vi "TSI Single Socket C-V Sweep SData Ver1.0.vi"(0 "Base Path":path=path "C:/Andy Tr/Wafer Level Measurement/WS102x", 1 "Package":string, 2 "Data In":string[][](array[string]), 3 "TP":string, 4 "Cyc":string, 5 "Cell":string, 7 "VDD To PGR OTP":string, 9 "Lot":string="Test", 10 "Index":i32, 11 "error in (no error)":errorcluster, 12 "Wafer":string="T8", 13 "X":string, 14 "Y":string) -> (15 "error out":errorcluster)   [LabVIEW 2017]
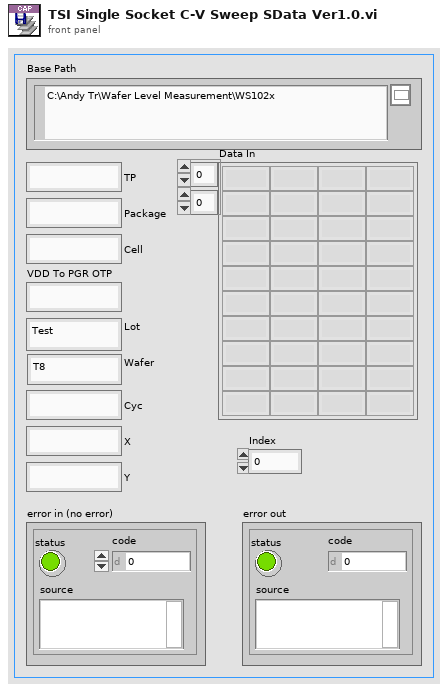
[diagram p1: front panel]
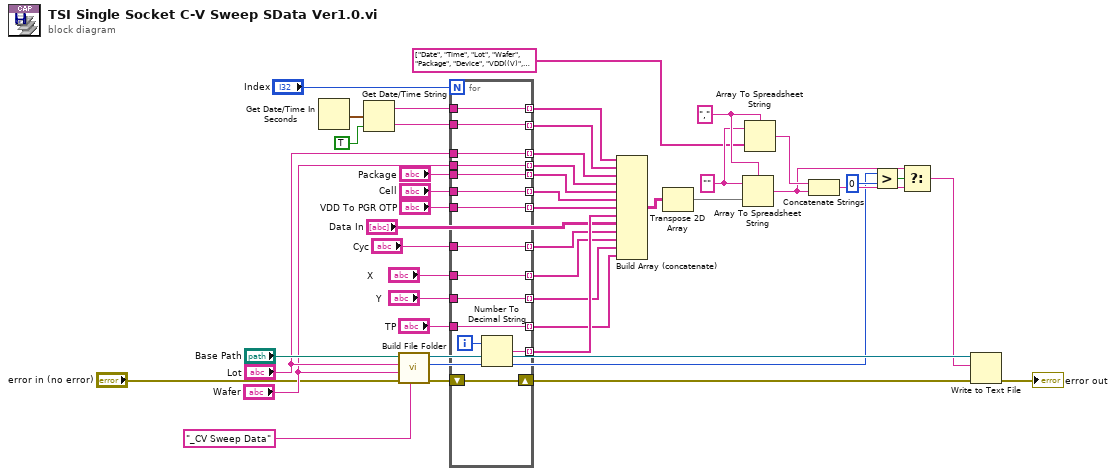
[diagram p0: block diagram]
diagram:
  w29 = "," ("delimiter (Tab)")
  w28 = "" ("format string")
  n1 = Get Date/Time In Seconds() -> (seconds since 1Jan1904=w41:timestamp)
  n2 = Get Date/Time String(seconds (now)=w41, want seconds? (F)=TRUE) -> (date string=w40:string, time string=w39:string)  [unwired: 1 in]
  n3 = call "Build File Folder.vi"("Data format"="_CV Sweep Data" ("File Name"), "error in (no error)"="error in (no error)", "Wafer"="Wafer", "Lot"="Lot", "TMN DC\\CAP Data Log File Path"="Base Path") -> ("error out"=w21:errorcluster, "size (in bytes)"=w26:i64, "Byte Stream File out"=w35:refnum<file>)  [unwired: 4 in]
  n4 = for {
    N: "Index" -> [_]
    tunnel: [w60] -> w9 mode=indexing
    tunnel: "VDD To PGR OTP" -> [w60]
    tunnel: "Package" -> [w59]
    tunnel: [w59] -> w13 mode=indexing
    tunnel: [w58] -> w12 mode=indexing
    tunnel: "Cell" -> [w58]
    tunnel: [w57] -> w17 mode=indexing
    tunnel: w40 -> [w57]
    tunnel: [w56] -> w16 mode=indexing
    tunnel: w39 -> [w56]
    tunnel: [w55] -> w15 mode=indexing
    tunnel: "Lot" -> [w55]
    tunnel: "Wafer" -> [w54]
    tunnel: [w54] -> w14 mode=indexing
    shift-right: [w53] -> w20
    shift-left: w21 -> [w53]
    tunnel: "TP" -> [w52]
    tunnel: [w52] -> w5 mode=indexing
    tunnel: [w50] -> w8 mode=indexing
    tunnel: "Cyc" -> [w49]
    tunnel: [w49] -> w6 mode=indexing
    tunnel: "X" -> [w48]
    tunnel: [w48] -> w3 mode=indexing
    tunnel: "Y" -> [w47]
    tunnel: [w47] -> w1 mode=indexing
    i -> [w51]
    n5 = Number To Decimal String(number=w51) -> (decimal integer string=w50:string)  [unwired: 1 in]
  }
  n6 = Build Array (concatenate)(w17, w16, w15, w14, w13, w12, w9, w8, "Data In", w6, w3, w1, w5) -> (w44:string[][])
  n7 = Transpose 2D Array(2D array=w44) -> (transposed array=w27:string[][])
  n8 = Array To Spreadsheet String(delimiter (Tab)=w29, array=w27, 3:w28) -> (spreadsheet string=w30:string)
  n9 = Array To Spreadsheet String(delimiter (Tab)=w29, array=string[] ["Date", "Time", "Lot", "Wafer", "Package", "Device", "VDD((V)", "Index", "I_Stdby(uA)", "CPV(V)", "Driver Name", "IDD_ON(uA)", "Cap(fF)", "DCAP(fF)", "Cycles", "X", "Y", "Test Program"] ("Header"), 3:w28) -> (spreadsheet string=w32:string)
  n10 = Concatenate Strings(w32, w30) -> (w31:string)
  n11 = Greater?(x=w26, y=i64 0) -> (0:w33:bool)
  n12 = Select(t=w30, s=w33, f=w31) -> (s? t:f=w25:string)
  n13 = Write to Text File(file (use dialog)=w35, text=w25, error in=w20) -> (error out=→"error out":errorcluster)  [unwired: 3 out]
